vi "Find Pupil1.vi"(11 "error in":errorcluster) -> (15 "error out":errorcluster)   [LabVIEW 2014]
uses:
  <vilib>/vision/NI_Vision_Development_Module.lvlib
panel:
  out "Image Out":T1(plugin-control)
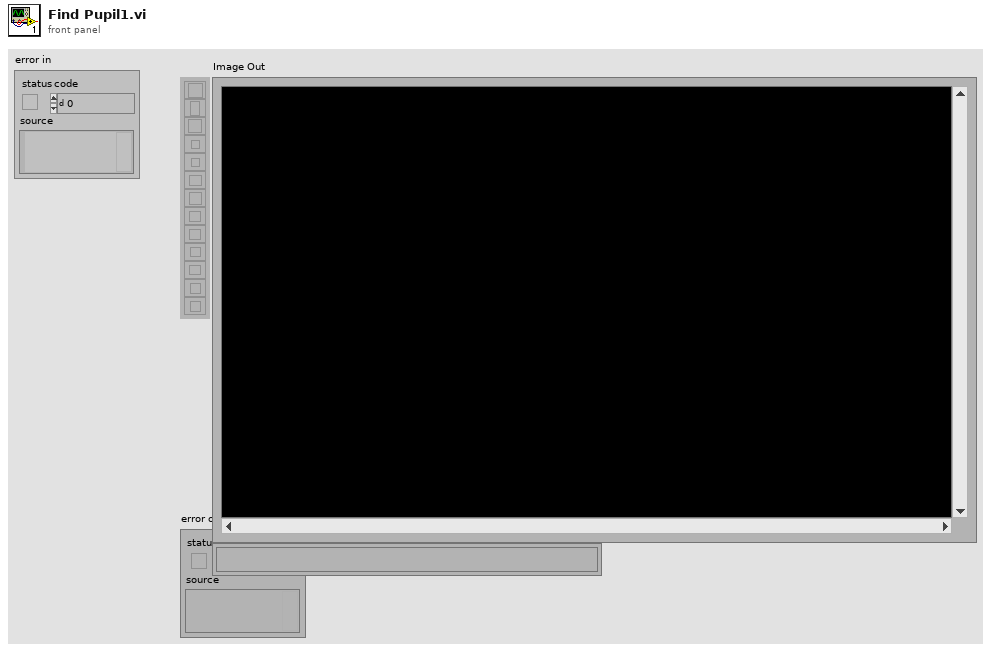
[diagram p1: front panel]
types:
  T1 = typedef "IMAQ Image.ctl" = refnum<image>
  T2 = cluster{"Left":i32, "Top":i32, "Right":i32, "Bottom":i32}
  T3 = typedef "Image Type" = u32
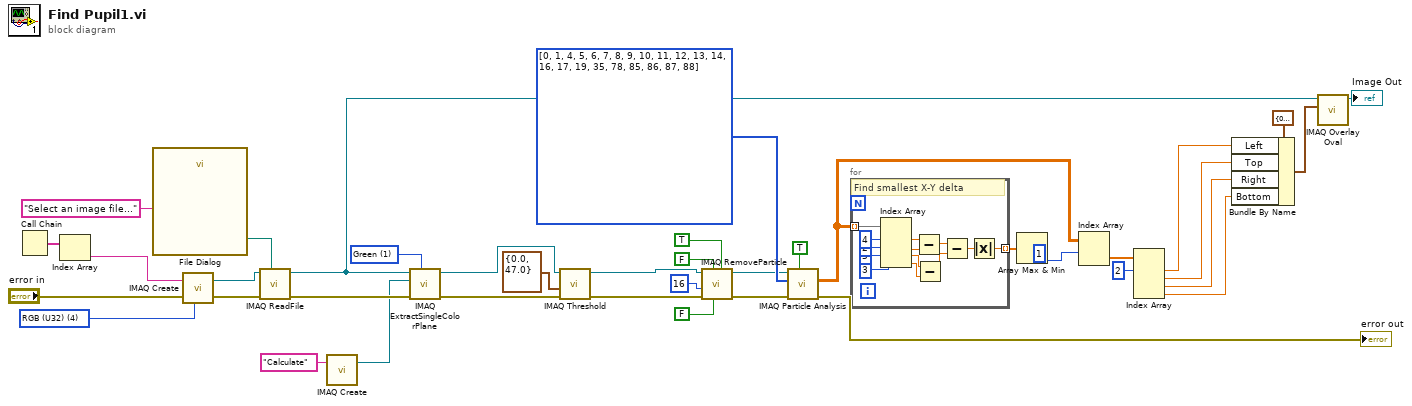
[diagram p0: block diagram]
diagram:
  (unwired) 1 ("index (row)")
  w19 = i32[] [0, 1, 4, 5, 6, 7, 8, 9, 10, 11, 12, 13, 14, 16, 17, 19, 35, 78, 85, 86, 87, 88] items=["Center of Mass X", "Center of Mass Y", "First Pixel X", "First Pixel Y", "Bounding Rect Left", "Bounding Rect Top", "Bounding Rect Right", "Bounding Rect Bottom", "Max Feret Diameter Start X", "Max Feret Diameter Start Y", "Max Feret Diameter End X", "Max Feret Diameter End Y", "Max Horiz. Segment Length Left", "Max Horiz. Segment Length Right", "Max Horiz. Segment Length Row", "-", "Bounding Rect Width", "Bounding Rect Height", "Bounding Rect Diagonal", "Perimeter", "Convex Hull Perimeter", "Holes' Perimeter", "Max Feret Diameter", "Equivalent Ellipse Major Axis", "Equivalent Ellipse Minor Axis", "Equivalent Ellipse Minor Axis (Feret)", "Equivalent Rect Long Side", "Equivalent Rect Short Side", "Equivalent Rect Diagonal", "Equivalent Rect Short Side (Feret)", "Average Horiz. Segment Length", "Average Vert. Segment Length", "Hydraulic Radius", "Waddel Disk Diameter", "-", "Area", "Holes' Area", "Particle & Holes' Area", "Convex Hull Area", "Image Area", "-", "Number of Holes", "Number of Horiz. Segments", "Number of Vert. Segments", "-", "Orientation", "Max Feret Diameter Orientation", "-", "% Area/Image Area", "% Area/(Particle & Holes' Area)", "Ratio of Equivalent Ellipse Axes", "Ratio of Equivalent Rect Sides", "-", "Elongation Factor", "Compactness Factor", "Heywood Circularity Factor", "Type Factor", "-", "Sum X", "Sum Y", "Sum XX", "Sum XY", "Sum YY", "Sum XXX", "Sum XXY", "Sum XYY", "Sum YYY", "-", "Moment of Inertia XX", "Moment of Inertia XY", "Moment of Inertia YY", "Moment of Inertia XXX", "Moment of Inertia XXY", "Moment of Inertia XYY", "Moment of Inertia YYY", "Norm. Moment of Inertia XX", "Norm. Moment of Inertia XY", "Norm. Moment of Inertia YY", "Norm. Moment of Inertia XXX", "Norm. Moment of Inertia XXY", "Norm. Moment of Inertia XYY", "Norm. Moment of Inertia YYY", "Hu Moment 1", "Hu Moment 2", "Hu Moment 3", "Hu Moment 4", "Hu Moment 5", "Hu Moment 6", "Hu Moment 7"] ("Pixel Measurements")
  w30 = 1 items=["Red", "Green", "Blue", "Hue", "Saturation", "Luminance", "Value", "Intensity"] ("Color Plane")
  w31 = T3 4 items=["Grayscale (U8)", "Grayscale (I16)", "Grayscale (SGL)", "Complex (CSG)", "RGB (U32)", "HSL (U32)", "RGB (U64)", "Grayscale (U16)"] ("Image Type")
  n1 = Call Chain() -> (call chain=w35:string[])
  n2 = Index Array(array=w35) -> (element=w34:string)  [unwired: 1 in]
  n3 = call "File Dialog"("prompt"="Select an image file...") -> ("selected path"=w32:path)  [unwired: 6 in, 8 out]
  n4 = call "IMAQ Create"("Image Name"=w34, "Image Type"=w31, "error in (no error)"="error in") -> ("New Image"=w38:T1, "error out"=w37:errorcluster)  [unwired: 1 in, 1 out]
  n5 = call "IMAQ ReadFile"("File Path"=w32, "error in (no error)"=w37, "Image"=w38) -> ("error out"=w39:errorcluster, "Image Out"=w11:T1)  [unwired: 2 in, 5 out]
  n6 = call "IMAQ Create"("Image Name"="Calculate") -> ("New Image"=w15:T1)  [unwired: 3 in, 2 out]
  n7 = call "IMAQ ExtractSingleColorPlane"("Color Plane"=w30, "error in (no error)"=w39, "Image Dst"=w15, "Image Src"=w11) -> ("error out"=w29:errorcluster, "Image Dst Out"=w27:T1)  [unwired: 6 out]
  n8 = call "IMAQ Threshold"("error in (no error)"=w29, "Range"=cluster{"Lower value":sgl, "Upper value":sgl} {"Lower value"=0.0, "Upper value"=47.0}, "Image Src"=w27) -> ("error out"=w26:errorcluster, "Image Dst Out"=w21:T1)  [unwired: 3 in, 4 out]
  n9 = call "IMAQ RemoveParticle"("Connectivity 4/8 (8)"=TRUE, "Low Pass/High Pass (Low)"=FALSE, "Square/Hexa (Square)"=FALSE, "error in (no error)"=w26, "Number of Erosion"=16, "Image Src"=w21) -> ("error out"=w20:errorcluster, "Image Dst Out"=w18:T1)  [unwired: 1 in, 3 out]
  n10 = call "IMAQ Particle Analysis"("Connectivity 4/8 (8)"=TRUE, "error in (no error)"=w20, "Pixel Measurements"=w19, "Image"=w18) -> ("error out"=→"error out":errorcluster, "Particle Measurements (Pixels)"=w1:dbl[][])  [unwired: 1 in, 5 out]
  n11 = for {
    tunnel: w1 -> [w52] mode=indexing
    tunnel: [w40] -> w3 mode=indexing
    # "Find smallest X-Y delta"
    n12 = Index Array(array=w52, index #1=4 ("index"), index #2=2 ("index"), index #3=5 ("index"), index #4=3 ("index")) -> (element #1=w48:dbl, element #2=w49:dbl, element #3=w45:dbl, element #4=w44:dbl)
    n13 = Subtract(x=w48, y=w49) -> (x-y=w43:dbl)
    n14 = Subtract(x=w45, y=w44) -> (x-y=w42:dbl)
    n15 = Subtract(x=w43, y=w42) -> (x-y=w41:dbl)
    n16 = Absolute Value(x=w41) -> (abs(x)=w40:dbl)
  }
  n17 = Array Max & Min(array=w3) -> (min index (indices)=w2:i32)  [unwired: 3 out]
  n18 = Index Array(array=w1, index (row)=w2) -> (element=w13:dbl[])  [unwired: 1 in]
  n19 = Index Array(array=w13, index #1=2 ("index")) -> (element #1=w7:dbl, element #2=w6:dbl, element #3=w5:dbl, element #4=w4:dbl)  [unwired: 3 in]
  n20 = Bundle By Name(cluster=T2 {"Left"=0, "Top"=0, "Right"=0, "Bottom"=0} ("Bounding Rectangle"), "Left"=w7, "Top"=w6, "Right"=w5, "Bottom"=w4) -> (w8:T2)
  n21 = call "IMAQ Overlay Oval"("Bounding Rectangle"=w8, "Image"=w11) -> ("Image Out"=→"Image Out":T1)  [unwired: 8 in, 1 out]
